vi "LabView360-3.vi"() -> ()   [LabVIEW 2017]
panel:
  in  "test":errorcluster caption="错误输出"
  out "输出簇":cluster{"布尔":bool, "数值":dbl, "字符串":string}
  out "字符串":string
  out "数值":dbl
  out "布尔":bool
  in  "簇":cluster{"布尔":bool, "数值":dbl, "字符串":string}
  out "last value":dbl
  out "auto-indexing":dbl[](array[numeric])
  out "result":i32
  in  "factor":i32
  out "result":dbl
  in  "fib":i32
  # "Cluster 是相当于绞线，可以将不同类型的数据打包成一个，或者作为 VI 的输入，解决连线板的端口不够的问题。"
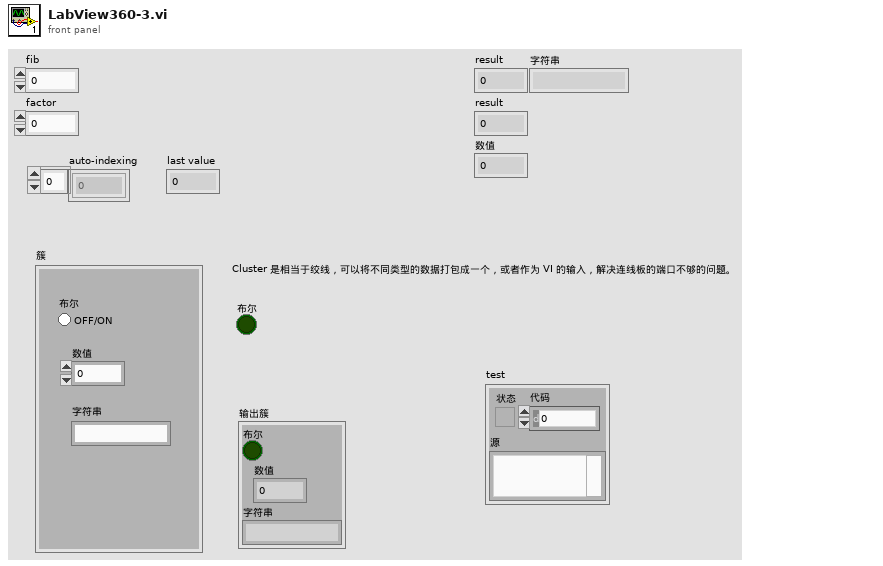
[diagram p1: front panel]
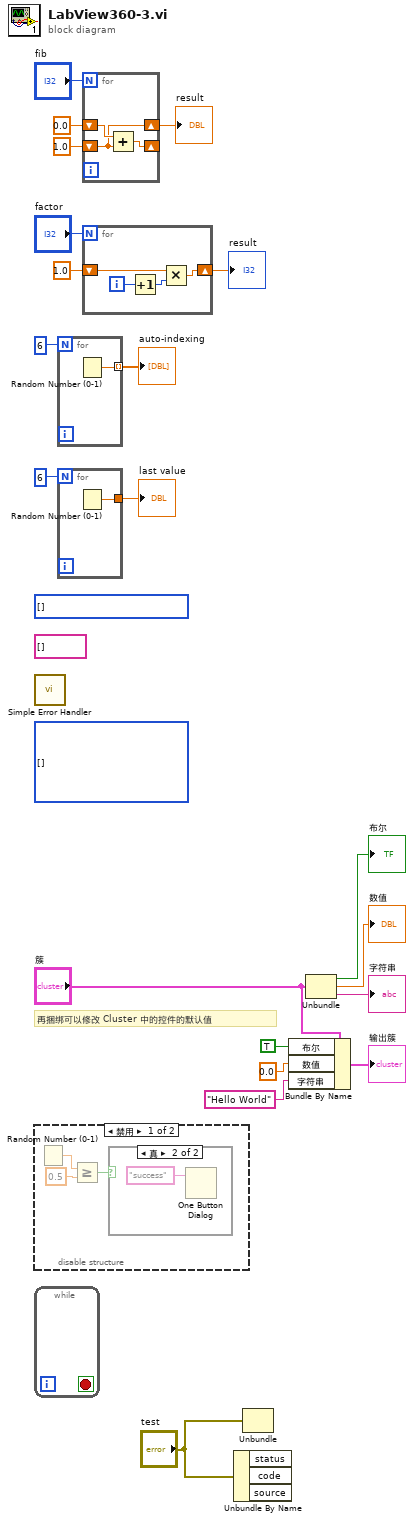
[diagram p0: block diagram]
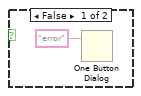
[diagram p2: hidden frame]
diagram:
  (unwired) i32[][] []
  (unwired) string[] []
  (unwired) i32[] []
  # "再捆绑可以修改 Cluster 中的控件的默认值"
  n1 = call <vilib>:"Simple Error Handler.vi"() -> ()  [unwired: 5 in, 5 out]
  n2 = disable-structure shown="禁用" {
    frame Disabled {
      n3 = Random Number (0-1)() -> (number: 0 to 1=w23:dbl)
      n4 = Greater Or Equal?(x=w23, y=0.5) -> (x >= y?=w22:bool)
      n5 = case shown="真" w22 {
        frame False {
          n6 = One Button Dialog(message="error" ("消息")) -> ()  [unwired: 1 in, 1 out]
        }
        frame True {
          n7 = One Button Dialog(message="success" ("消息")) -> ()  [unwired: 1 in, 1 out]
        }
      }
    }
    frame Enabled {
    }
  }
  n8 = while {
    stop <- _ stop-if-true
  }
  n9 = for {
    N: 6 -> [_]
    tunnel: [w26] -> w12 mode=indexing
    n10 = Random Number (0-1)() -> (number: 0 to 1=w26:dbl)
  }
  "auto-indexing" <- w12
  n11 = for {
    N: 6 -> [_]
    tunnel: [w27] -> w10
    n12 = Random Number (0-1)() -> (number: 0 to 1=w27:dbl)
  }
  "last value" <- w10
  n13 = for {
    N: "fib" -> [_]
    shift-right: [w28] -> w17
    shift-left: 0.0 -> [w30]
    shift-right: [w29] -> _
    shift-left: 1.0 -> [w28]
    n14 = Add(x=w30, y=w28) -> (x+y=w29:dbl)
  }
  "result" <- w17
  n15 = for {
    N: "factor" -> [_]
    shift-right: [w33] -> w15
    shift-left: 1.0 -> [w34]
    i -> [w31]
    n16 = Increment(x=w31) -> (x+1=w32:i32)
    n17 = Multiply(x=w34, y=w32) -> (x*y=w33:dbl)
  }
  "result" <- w15
  n18 = Unbundle By Name("test") -> ()  [unwired: 3 out]
  n19 = Unbundle("test") -> ()  [unwired: 3 out]
  n20 = Bundle By Name(cluster="簇", "布尔"=TRUE, "数值"=0.0, "字符串"="Hello World") -> (→"输出簇":cluster{"布尔":bool, "数值":dbl, "字符串":string})
  n21 = Unbundle("簇") -> ("布尔"=→"布尔":bool, "数值"=→"数值":dbl, "字符串"=→"字符串":string)
